vi "Load New Launcher.vi"(7 "Plugin Loader Path Override":path, 8 "error in (no error)":errorcluster, 9 "Loader Name Override":string, 10 "Loader Load Info":T1, 11 "CIFPluginManager in":refnum<class "CIFPluginManager.lvclass">) -> (0 "error out":errorcluster)   [LabVIEW 2021, in "CIFPluginManager.lvclass"]
uses:
  CIFPluginManager.lvclass
  typedef/Loader Load Command.ctl
  typedef/Loader Type.ctl
  CIFPluginManager.lvclass/CIFPluginManager.ctl
  CIFUtilities/CIFConfigurationFile/typedef/Location Type.ctl
  CIFUtilities/CIFConfigurationFile/CIF Configuration File Location.vi
  Engine Launch/CIF Engine Launch.lvlib
  <vilib>/CIF Foundation/CIF Utilities/Time/Time_CIF_U.lvlib
  CIFUtilities/CIFConfigurationFile/CIF Configuration File.lvlib
  CIFCore/Common/CIFCoreCommon.lvlib
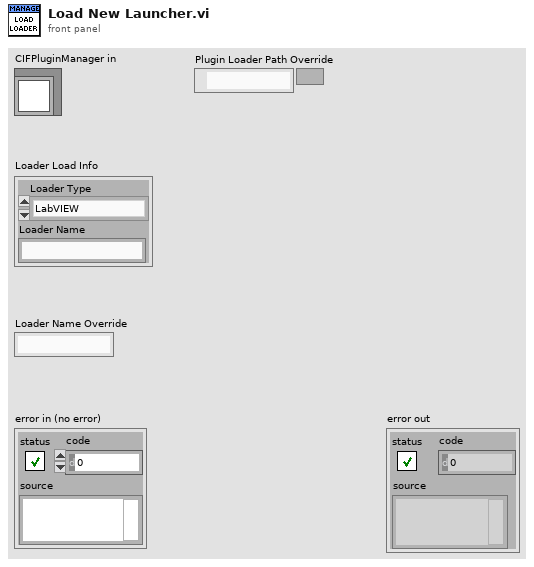
[diagram p1: front panel]
types:
  T1 = typedef "CIFPluginManager.lvclass/Loader Load Command.ctl" = cluster{"Loader Type":T2, "Loader Name":string}
  T2 = typedef "CIFPluginManager.lvclass/Loader Type.ctl" = enum16{"LabVIEW"}
  T3 = typedef "CIF Configuration File.lvlib/Location Type.ctl" = enum16{"Config File", "Manager", "Protos", "Plugins", "UI Plugins", "Logs", "Orchestrations", "Loaders"}
  T4 = typedef "CIFPluginManager.lvclass/Loader Map.ctl" = map{string, T5}
  T5 = typedef "CIFPluginManager.lvclass/Loaders.ctl" = cluster{"Loader Type":T2, "grpc_port":i32, "pid":u32, "gRPC ID":T6, "Load Timestamp":i64, "Unloading":bool, "Ready for removal":bool, "Unload Timestamp":i64}
  T6 = typedef "grpc-lvsupport-release.lvlib/grpcId.ctl" = u64
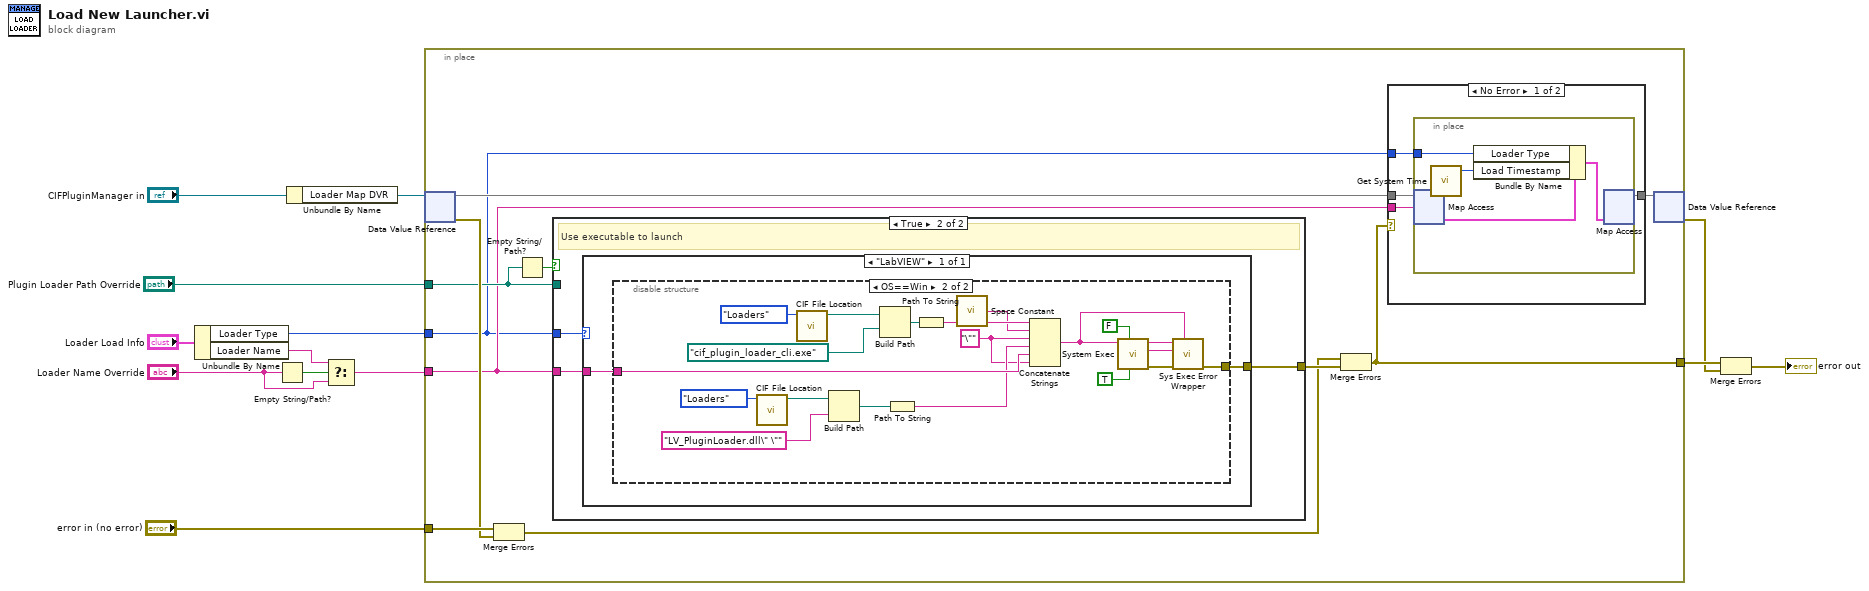
[diagram p0: block diagram]
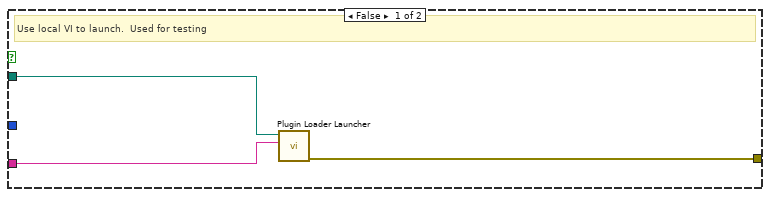
[diagram p3: hidden frame]
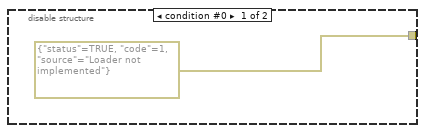
[diagram p4: hidden frame]
diagram:
  n1 = Unbundle By Name("Loader Load Info") -> ("Loader Type"=w1:T2, "Loader Name"=w4:string)
  n2 = Empty String/Path?(string/path="Loader Name Override") -> (empty?=w6:bool)
  n3 = Unbundle By Name("CIFPluginManager in") -> ("Loader Map DVR"=w11:refnum<data-value>)
  n4 = Select(t=w4, s=w6, f="Loader Name Override") -> (s? t:f=w3:string)
  n5 = in-place {
    in-place-border: "error in (no error)" -> [w24]
    in-place-border: [w15] -> w10
    in-place-border: w3 -> [w17]
    in-place-border: "Plugin Loader Path Override" -> [w22]
    in-place-border: w1 -> [w14]
    n6 = in-place-dvr #1(w11) -> (w18:T4, w23:errorcluster)
    n7 = Merge Errors(w24, w23) -> (w19:errorcluster)
    n8 = Empty String/Path?(string/path=w22) -> (empty?=w21:bool)
    n9 = case shown="True" w21 {
      tunnel: w22 -> [w36 _]
      tunnel: [w35 w38] -> w20
      tunnel: w17 -> [w34 w39]
      tunnel: w14 -> [_ w37]
      frame False {
        # "Use local VI to launch.  Used for testing"
        n10 = call "Plugin Loader Launcher.vi"("Loader Name Override"=w34, "Plugin Loader Path Override"=w36) -> ("error out"=w35:errorcluster)  [unwired: 9 in]
      }
      frame True {
        # "Use executable to launch"
        n11 = case shown="\"LabVIEW\"" w37 {
          tunnel: w39 -> [w41]
          tunnel: [w40] -> w38
          frame "LabVIEW" {
            n12 = disable-structure shown="OS==Win" {
              disable-tunnel: w41 -> [_ w52]
              disable-tunnel: [errorcluster {"status"=TRUE, "code"=1, "source"="Loader not implemented"} ("error out") w46] -> w40
              frame condition #0 {
              }
              frame condition #1 (active) {
                w48 = "\"" ("Loader Name Override")
                n13 = call "CIF File Location.vi"("LocationType"=Location_Type."Loaders") -> ("Location"=w54:path)  [unwired: 10 in]
                n14 = call "CIF File Location.vi"("LocationType"=Location_Type."Loaders") -> ("Location"=w58:path)  [unwired: 10 in]
                n15 = Build Path(base path=w54, name or relative path="LV_PluginLoader.dll\" \"" ("Loader Name Override")) -> (appended path=w51:path)
                n16 = Build Path(base path=w58, name or relative path=path "cif_plugin_loader_cli.exe") -> (appended path=w62:path)
                n17 = Path To String(path=w51) -> (string=w50:string)
                n18 = Path To String(path=w62) -> (string=w61:string)
                n19 = call <vilib>:"Space Constant.vi"() -> ("String"=w49:string)
                n20 = Concatenate Strings(w61, w49, w48, w50, w52, w48) -> (w43:string)
                n21 = call <vilib>:"System Exec.vi"("run minimized? (F)"=TRUE, "wait until completion? (T)"=FALSE, "command line"=w43) -> ("error out"=w47:errorcluster, "standard error"=w45:string, "standard output"=w44:string)  [unwired: 5 in, 1 out]
                n22 = call "Sys Exec Error Wrapper.vi"("command line"=w43, "error in (no error)"=w47, "standard error"=w45, "standard output"=w44) -> ("error out"=w46:errorcluster)  [unwired: 7 in]
              }
            }
          }
        }
      }
    }
    n23 = Merge Errors(w19, w20) -> (w15:errorcluster)
    n24 = case shown="No Error" w15 {
      tunnel: w18 -> [w28 w33]
      tunnel: w17 -> [w27 _]
      tunnel: [w26 w33] -> w16
      tunnel: w14 -> [w25 _]
      frame No Error {
        n25 = in-place {
          in-place-border: w25 -> [w29]
          n26 = in-place-map #2(w28, w27) -> (w32:T5)  [unwired: 1 in, 1 out]
          n27 = call <vilib>:"Get System Time.vi"() -> ("Time (ns)"=w31:i64)  [unwired: 5 in]
          n28 = Bundle By Name(cluster=w32, "Loader Type"=w29, "Load Timestamp"=w31) -> (w30:T5)
          n29 = in-place-map #2(w30) -> (w26:T4)  [unwired: 1 in, 2 out]
        }
      }
      frame Error {
      }
    }
    n30 = in-place-dvr #1(w16) -> (w9:errorcluster)  [unwired: 1 out]
  }
  n31 = Merge Errors(w10, w9) -> (→"error out":errorcluster)
